vi "Save to file with time stamp.vi"(0 "T in":dbl, 1 "number of data sample":u64, 2 "Average in":dbl, 3 "d/dt in":dbl, 4 "refnum file":refnum<file>, 5 "error in":errorcluster) -> (15 "number of data sample out":u64, 19 "error out":errorcluster)   [LabVIEW 2013]
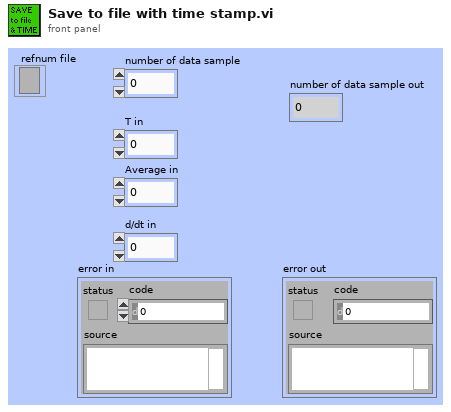
[diagram p1: front panel]
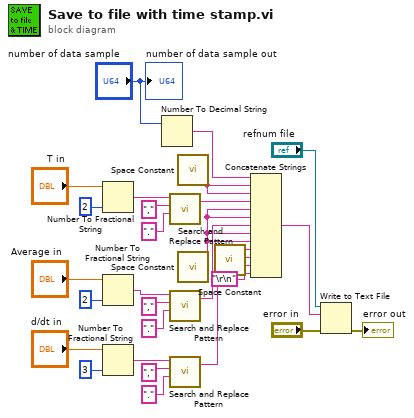
[diagram p0: block diagram]
diagram:
  n1 = Number To Fractional String(number="T in", precision (6)=i16 2) -> (F-format string=w22:string)  [unwired: 2 out]
  n2 = Number To Fractional String(number="Average in", precision (6)=i16 2) -> (F-format string=w16:string)  [unwired: 2 out]
  n3 = Number To Fractional String(number="d/dt in", precision (6)=i16 3) -> (F-format string=w11:string)  [unwired: 2 out]
  n4 = Number To Decimal String(number="number of data sample") -> (decimal integer string=w2:string)  [unwired: 1 out]
  n5 = call <vilib>:"Search and Replace Pattern.vi"("string"=w22, "regular expression (\"\")"="," ("regular expression (\"\")"), "replace string (\"\")"="." ("replace string (\"\")")) -> ("result string"=w8:string)  [unwired: 3 out]
  n6 = call <vilib>:"Search and Replace Pattern.vi"("string"=w16, "regular expression (\"\")"="," ("regular expression (\"\")"), "replace string (\"\")"="." ("replace string (\"\")")) -> ("result string"=w7:string)  [unwired: 3 out]
  n7 = call <vilib>:"Search and Replace Pattern.vi"("string"=w11, "regular expression (\"\")"="," ("regular expression (\"\")"), "replace string (\"\")"="." ("replace string (\"\")")) -> ("result string"=w6:string)  [unwired: 3 out]
  n8 = call <vilib>:"Space Constant.vi"() -> ("String"=w1:string)
  n9 = call <vilib>:"Space Constant.vi"() -> ("String"=w3:string)
  n10 = call <vilib>:"Space Constant.vi"() -> ("String"=w5:string)
  n11 = Concatenate Strings(w2, w1, w1, w8, w3, w3, w7, w3, w3, w6, w5, w5, "\r\n") -> (w23:string)
  n12 = Write to Text File(file (use dialog)="refnum file", text=w23, error in="error in") -> (error out=→"error out":errorcluster)  [unwired: 3 out]
  "number of data sample out" <- "number of data sample"
